vi "Write Action to File.vi"(0 "role":string, 1 "action_code":cluster{i32, i32, i32}) -> ()   [LabVIEW 2025]
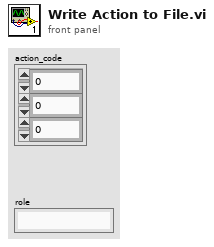
[diagram p1: front panel]
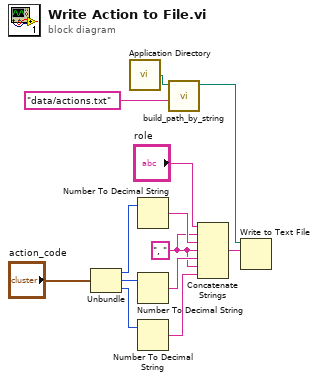
[diagram p0: block diagram]
diagram:
  w6 = ", " ("string")
  n1 = Unbundle("action_code") -> (w7:i32, w9:i32, w10:i32)
  n2 = call <vilib>:"Application Directory.vi"() -> ("Application Directory"=w1:path)
  n3 = Number To Decimal String(number=w7) -> (decimal integer string=w8:string)  [unwired: 1 in]
  n4 = Number To Decimal String(number=w9) -> (decimal integer string=w12:string)  [unwired: 1 in]
  n5 = Number To Decimal String(number=w10) -> (decimal integer string=w11:string)  [unwired: 1 in]
  n6 = call "build_path_by_string.vi"("String"="data/actions.txt", "base path"=w1) -> ("appended path"=w3:path)  [unwired: 9 in]
  n7 = Concatenate Strings("role", w6, w8, w6, w12, w6, w11) -> (w13:string)
  n8 = Write to Text File(file (use dialog)=w3, text=w13) -> ()  [unwired: 2 in, 3 out]
